vi "Uploading 128 file.vi"(8 "error in (no error)":errorcluster, 10 ".128 file Path":path=path "E:/LCU6331 test/Procedure2/RFID_m645_Prodtest_LCU6331.128" caption="Path", 11 "VISA resource name":refnum<visa-resource-name>="COM8") -> (0 "error out":errorcluster, 1 "Error Lin":i32, 2 "Pass?":bool, 3 "VISA resource name out":refnum<visa-resource-name>)   [LabVIEW 2009]
uses:
  <vilib>/Instr/_visa.llb/VISA Configure Serial Port (Instr).vi
panel:
  out "Numeric":i32
  out "String":string
  out "Uploading":u8(slide) caption="Slide" scale=0.0..79.0
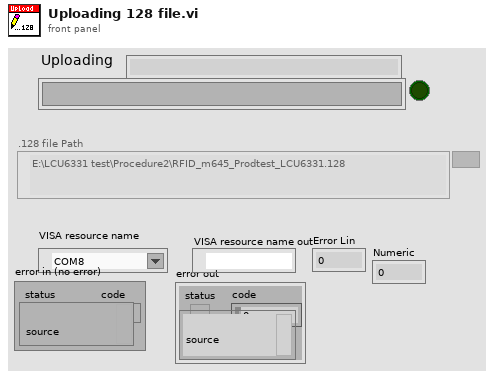
[diagram p1: front panel]
types:
  T1 = enum16{"Start-up", "change baud rate", "set 218 file", "finish"}
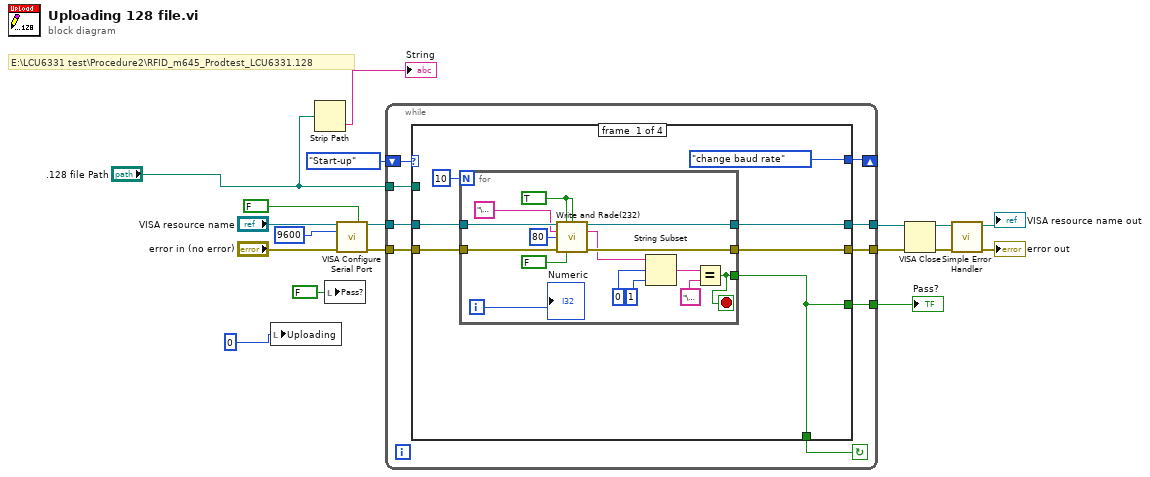
[diagram p0: block diagram]
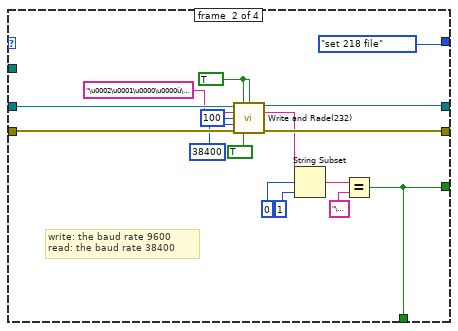
[diagram p2: hidden frame]
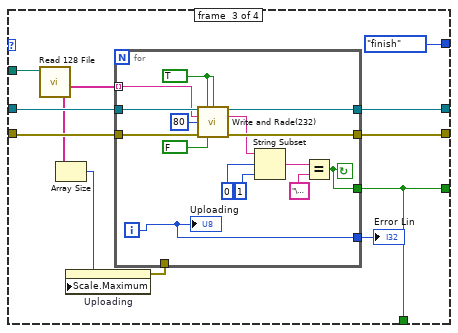
[diagram p3: hidden frame]
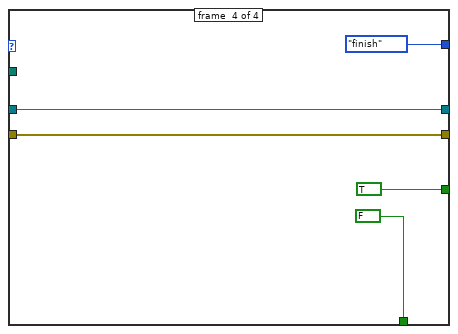
[diagram p4: hidden frame]
diagram:
  # "E:\\LCU6331 test\\Procedure2\\RFID_m645_Prodtest_LCU6331.128"
  n1 = local write "Uploading"(u8 0 ("Slide")) -> ()
  n2 = Strip Path(path=".128 file Path") -> (name=→"String":string)  [unwired: 1 out]
  n3 = local write "Pass?"(FALSE ("Pass?")) -> ()
  n4 = call-poly "VISA Configure Serial Port"("VISA resource name"="VISA resource name", "Enable Termination\nChar (T)"=FALSE ("Enable Termination\nChar (T)"), "baud rate (9600)"=u32 9600, "error in (no error)"="error in (no error)") -> ("VISA resource name out"=w7:refnum<visa-resource-name>, "error out"=w9:errorcluster)  [unwired: 3 in, 7 out]
  n5 = while {
    shift-right: [w24] -> _
    shift-left: T1."Start-up" -> [w25]
    tunnel: w7 -> [w22]
    tunnel: w9 -> [w21]
    tunnel: [w20] -> w11
    tunnel: [w19] -> w10
    tunnel: [w18] -> w6
    tunnel: ".128 file Path" -> [w17]
    stop <- w23 continue-if-true
    n6 = case shown="\"change baud rate\"" w25 {
      tunnel: [T1."change baud rate" T1."set 218 file" T1."finish" T1."finish"] -> w24
      tunnel: [w27 w49 w65 FALSE] -> w23
      tunnel: w22 -> [w31 w62 w73 w93]
      tunnel: w21 -> [w29 w61 w72 w92]
      tunnel: [w30 w60 w71 w93] -> w20
      tunnel: [w28 w59 w70 w92] -> w19
      tunnel: [w27 w49 w65 TRUE] -> w18
      tunnel: w17 -> [_ _ w66 _]
      frame #0 {
        n7 = for {
          N: 10 -> [_]
          tunnel: w31 -> [w47]
          tunnel: [w46] -> w30
          tunnel: w29 -> [w45]
          tunnel: [w44] -> w28
          tunnel: [w34] -> w27
          i -> [w33]
          stop <- w34 stop-if-true
          w37 = TRUE ("write")
          n8 = call "Write and Rade(232).vi"("VISA resource name in"=w47, "write"=w37, "read"=w37, "string to write"="\u0016", "ms delay"=u32 80 ("millisecond multiple"), "error in"=w45, "change baud rate(read)"=FALSE ("change baud rate")) -> ("VISA resource name out"=w46:refnum<visa-resource-name>, "read string"=w39:string, "error out"=w44:errorcluster)  [unwired: 1 in, 5 out]
          n9 = String Subset(string=w39, offset (0)=0, length (rest)=1 ("length (rest)")) -> (substring=w41:string)
          n10 = Equal?(x=w41, y="\u0006") -> (x = y?=w34:bool)
          "Numeric" <- w33
        }
      }
      frame #1 {
        w53 = TRUE ("write")
        # "write: the baud rate 9600\nread: the baud rate 38400"
        n11 = call "Write and Rade(232).vi"("VISA resource name in"=w62, "write"=w53, "read"=w53, "string to write"="\u0002\u0001\u0000\u0000ù\rù", "ms delay"=u32 100 ("millisecond multiple"), "baud rate(read)"=u32 38400 ("baud rate"), "error in"=w61, "change baud rate(read)"=TRUE ("change baud rate")) -> ("VISA resource name out"=w60:refnum<visa-resource-name>, "read string"=w54:string, "error out"=w59:errorcluster)  [unwired: 5 out]
        n12 = String Subset(string=w54, offset (0)=0, length (rest)=1 ("length (rest)")) -> (substring=w56:string)
        n13 = Equal?(x=w56, y="\u0006") -> (x = y?=w49:bool)
      }
      frame #2 {
        n14 = call "Read 128 File.vi"("Path"=w66) -> ("输出数组"=w69:string[])  [unwired: 1 in, 9 out]
        n15 = Array Size(array=w69) -> (size(s)=w68:i32)
        n16 = property on="Uploading" class="Slide (strict)"("Scale.Maximum"=w68) -> (error out=w67:errorcluster)  [unwired: 2 in, 1 out]
        n17 = for {
          tunnel: w73 -> [w89]
          tunnel: w72 -> [w88]
          tunnel: [w87] -> w71
          tunnel: [w86] -> w70
          tunnel: w69 -> [w78] mode=indexing
          tunnel: [w77] -> w65
          tunnel: w67 -> [_]
          tunnel: [w75] -> w64
          i -> [w75]
          stop <- w77 continue-if-true
          w80 = TRUE ("write")
          n18 = call "Write and Rade(232).vi"("VISA resource name in"=w89, "write"=w80, "read"=w80, "string to write"=w78, "ms delay"=u32 80 ("millisecond multiple"), "error in"=w88, "change baud rate(read)"=FALSE) -> ("VISA resource name out"=w87:refnum<visa-resource-name>, "read string"=w81:string, "error out"=w86:errorcluster)  [unwired: 1 in, 5 out]
          n19 = String Subset(string=w81, offset (0)=0, length (rest)=1 ("length (rest)")) -> (substring=w83:string)
          n20 = Equal?(x=w83, y="\u0006") -> (x = y?=w77:bool)
          "Uploading" <- w75
        }
        "Error Lin" <- w64
      }
      frame #3 {
      }
    }
  }
  "Pass?" <- w6
  "VISA resource name out" <- w11
  n21 = VISA Close(VISA resource name=w11, error in (no error)=w10) -> (error out=w12:errorcluster)
  n22 = call <vilib>:"Simple Error Handler.vi"("error in (no error)"=w12) -> ("error out"=→"error out":errorcluster)  [unwired: 1 in, 7 out]
